vi "Enable Subsystem.vi"(10 "regular expression":string, 11 "List of Device Names to check against what you expect":string[](array[string])) -> (2 "Enable?":bool)   [LabVIEW 2018]
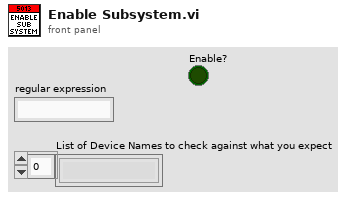
[diagram p1: front panel]
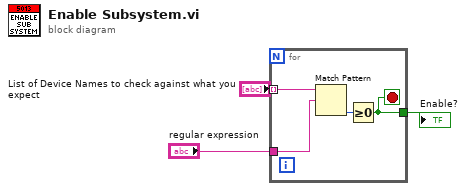
[diagram p0: block diagram]
diagram:
  n1 = for {
    tunnel: "List of Device Names to check against what you expect" -> [w7] mode=indexing
    tunnel: "regular expression" -> [w6]
    tunnel: [w4] -> w1
    stop <- w4 stop-if-true
    n2 = Match Pattern(string=w7, regular expression=w6) -> (offset past match=w5:i32)  [unwired: 1 in, 3 out]
    n3 = Greater Or Equal To 0?(x=w5) -> (x >= 0?=w4:bool)
  }
  "Enable?" <- w1
